vi "DPOreadRaise.vi"(3 "错误输入（无错误）":errorcluster, 5 "VISA资源名称":refnum<visa-resource-name>) -> (0 "错误输出":errorcluster, 1 "上升沿时间":dbl, 2 "VISA资源名称输出":refnum<visa-resource-name>)   [LabVIEW 2018]
uses:
  <instrlib>/Tektronix DPO MSO 2000 4000 Series/Tektronix DPO MSO 2000 4000 Series.lvlib
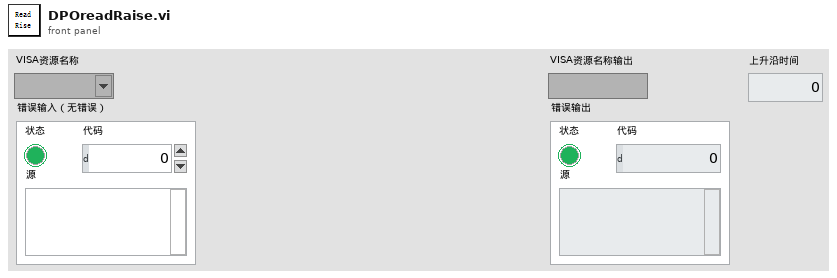
[diagram p1: front panel]
types:
  T1 = typedef "IMAQ Image.ctl" = refnum<image>
  T2 = cluster{"示波器":cluster{"Channel (0:Channel 1)":enum16{"Channel 1", "Channel 2", "Channel 3", "Channel 4"}, "电压范围":dbl, "触发电压":dbl, "时间范围":dbl, " 示波器VISA":refnum<visa-resource-name>, "时间范围 标签":u64, "电压范围 标签":u64}, "光谱仪":cluster{"Channel (0:Channel 1)":enum16{"Channel 1", "Channel 2", "Channel 3", "Channel 4"}, "电压范围":u64, "触发电压":u64, "时间范围":u64}, " 近场相机":cluster{"曝光时间":i32, "模拟增益":i32, "控制套接字":i32, "IP 地址":string, " 采集套接字":i32, "  版本号":i32, "ImageData":T1, "  增益最大":i32, "  增益最小":i32, " 曝光最大":i32, " 曝光最小":i32, " 帧速":i32, " 同步切换":i32, "  曝光缩放":i32}, " 偏振仪":cluster{"电压范围":u64, "触发电压":u64, "时间范围":u64, "波长范围":enum16{"可见光 400-700nm", "近红外 700-1100nm"}}, " 功率计":cluster{"通道":enum16{"Channel 1", "Channel 2"}, "工作波长":u32, "单位":u64, "时间范围":u64, "IP地址":string, "端口":u32}, "能量计":cluster{"通道":enum16{"Channel 1", "Channel 2"}, "工作波长":u32, "单位":u64, "时间范围":u64, "IP地址":string, "端口":u32, "能量计量程":enum16{"200uJ", "20uJ", "2uJ", "200nJ"}}, "电机":cluster{"Channel (0:Channel 1)":enum16{"Channel 1", "Channel 2", "Channel 3", "Channel 4"}, "电压范围":u64, "触发电压":u64, "时间范围":u64}, " 远场相机":cluster{"曝光时间":i32, "模拟增益":i32, "控制套接字":i32, "IP 地址":string, " 采集套接字":i32, "  版本号":i32, "ImageData":T1, "  增益最大":i32, "  增益最小":i32, " 曝光最大":i32, " 曝光最小":i32, " 帧速":i32, " 同步切换":i32, "  曝光缩放":i32}}
  T3 = enum16{"Channel 1", "Channel 2", "Channel 3", "Channel 4"}
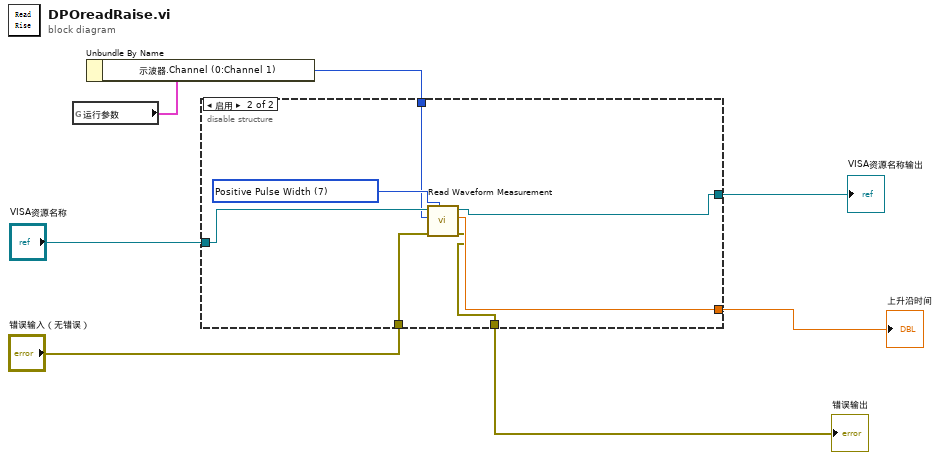
[diagram p0: block diagram]
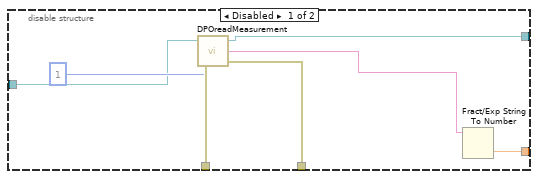
[diagram p2: hidden frame]
diagram:
  n1 = global read "参数.vi" "运行参数"() -> (w2:T2)
  n2 = Unbundle By Name(w2) -> ("示波器.Channel (0:Channel 1)"=w1:T3)
  n3 = disable-structure shown="启用" {
    disable-tunnel: "错误输入（无错误）" -> [w14 w19]
    disable-tunnel: [w13 w16] -> w6
    disable-tunnel: [w10 w17] -> w5
    disable-tunnel: "VISA资源名称" -> [w9 w21]
    disable-tunnel: [w8 w18] -> w3
    disable-tunnel: w1 -> [_ w15]
    frame Disabled {
      n4 = call "DPOreadMeasurement.vi"("错误输入（无错误）"=w14, "通道"=u8 1, "VISA资源名称"=w9) -> ("错误输出"=w13:errorcluster, "data out"=w11:string, "VISA资源名称输出"=w8:refnum<visa-resource-name>)
      n5 = Fract/Exp String To Number(string=w11) -> (number=w10:dbl)  [unwired: 3 in, 1 out]
    }
    frame Enabled {
      w20 = 7 items=["Period", "Frequency", "Delay", "Rise Time", "Fall Time", "Positive Duty Cycle", "Negative Duty Cycle", "Positive Pulse Width", "Negative Pulse Width", "Burst Width", "Phase", "Positive Overshoot", "Negative Overshoot", "Vpp", "Amplitude", "Voltage High", "Voltage Low", "Voltage Max", "Voltage Min", "Voltage Mean", "Voltage Mean (cycle)", "Voltage RMS", "Voltage RMS (cycle)", "Area", "Cycle Area", "Positive Edge Count", "Negative Edge Count", "Positive Pulse Count", "Negative Pulse Count", "Total Overshoot"] ("Measurement Function (0: Period)")
      n6 = call <instrlib>:"Read Waveform Measurement.vi"("Measurement Function (0: Period)"=w20, "error in (no error)"=w19, "Channel (0: Channel 1)"=w15, "VISA resource name"=w21) -> ("error out"=w16:errorcluster, "Measurement Value"=w17:dbl, "VISA resource name out"=w18:refnum<visa-resource-name>)  [unwired: 5 in]
    }
  }
  "错误输出" <- w6
  "上升沿时间" <- w5
  "VISA资源名称输出" <- w3
